vi "Restore to Defaults.vi"(6 "User interface enqueuer":refnum<class "Message Enqueuer.lvclass">, 7 "Rack Number":string, 8 "error in":errorcluster, 9 "JSON Variant Clusters":T1, 10 "JSON path cluster":T2, 11 "Part Name in":string) -> (0 "error out":errorcluster, 2 "Algo JSON variant":variant, 3 "RC JSON variant":variant)   [LabVIEW 2019, in "ZenGage v3.0 UI.lvclass"]
uses:
  ZenGage v3.0 UI.lvclass
  User Interface Messages/User Interface messages/Display Popup Msg/DisplayPopup_UI.lvclass
  Common/Controls/Pop-up Input.ctl
  <vilib>/Utility/miscctls.llb/LVPoint32TypeDef.ctl
  Type Definitions/Edit tolerance settings/Rack Selection.ctl
  <vilib>/ActorFramework/Message Enqueuer/Message Enqueuer.lvclass
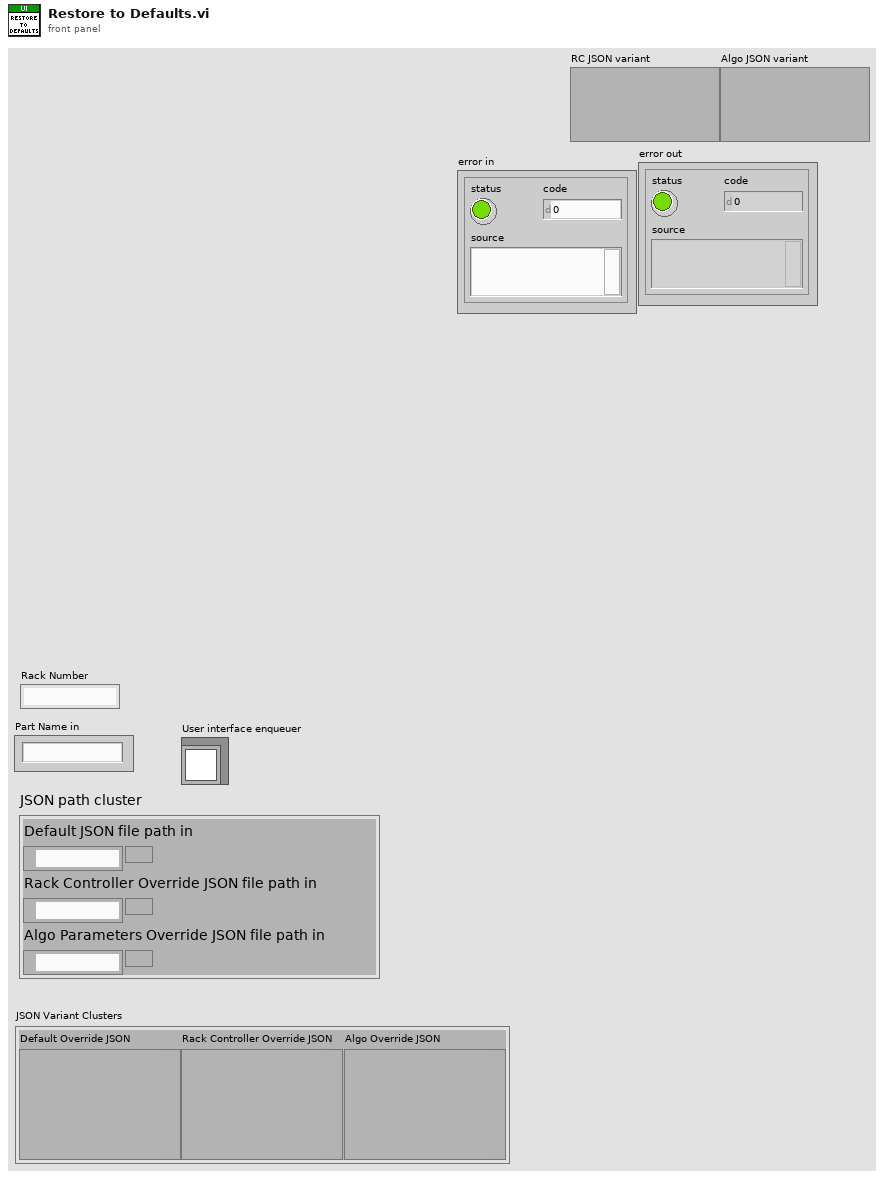
[diagram p1: front panel]
types:
  T1 = cluster{"Default Override JSON":variant, "Rack Controller Override JSON":variant, "Algo Override JSON":variant}
  T2 = cluster{"Default JSON file path in":path, "Rack Controller Override JSON file path in":path, "Algo Parameters Override JSON file path in":path}
  T3 = typedef "ZenGage v3.0 UI.lvclass/Rack Selection.ctl" = enum16{"Both Racks", "Rack 2", "Rack 1"}
  T4 = typedef "LVPoint32TypeDef.ctl" = cluster{"Horizontal":i32, "Vertical":i32}
  T5 = cluster{"Measurement Values":string[][], "Cluster of Limits":cluster{"LSL":dbl, "USL":dbl, "LCL":dbl, "UCL":dbl}, "Rack Selection":T3, "M and N Array":cluster{"M1":u64, "M2":u64, "N1":u64, "N2":u64}[], "Ticked Measurement Index":u32[], "Measurements Enabled":bool[], "Current Active Position":T4, "Current ticked measurement":dbl}
  T6 = typedef "Pop-up Input.ctl" = cluster{"Pop-up Type":enum16{"Open Logo Display", "Close Logo Display", "Open Loading Bar", "Close Loading Bar", "Open Alert Display", "Close Alert Display", "One button dialog box", "Two button dialog box", "User Authentication"}, "Title":string, "Message":string, "Button 1 Text":string, "Button 2 Text":string, "Show Close? T/F":bool, "Title Blink? T/F":bool, "Title Blink Colour":u32}
  T7 = cluster{"Measurement Values":string[][], "Enabled Disable Array":bool[]}
  T8 = cluster{"Name":string, "ImageStreams":cluster{"ThreadName":string, "RackEnable":bool, "ThreadId":dbl, "RackId":dbl, "DifferenceParameter":dbl, "SplitCameraIDs":i32[], "ImagingViews":cluster{"ViewName":string, "ViewEnable":bool, "ImageID":dbl, "CameraID":dbl, "CalibrationFilePath":string, "CalibImageFormat":string, "ReferenceCoordSystem":cluster{"Method":cluster{"Algo":string, "BaseReference":cluster{"OriginX":dbl, "OriginY":dbl, "Angle":dbl, "AxisReference":dbl}}, "ROI":cluster{"ROI":cluster{"Left":dbl, "Top":dbl, "Right":dbl, "Bottom":dbl, "Rotation":dbl}, "EdgeOptions":cluster{"EdgePolarity":dbl, "KernelSize":dbl, "Width":dbl, "MinimumEdgeStrength":dbl, "InterpolationType":dbl, "DataProcessingMethod":dbl}, "LineOptions":cluster{"NumberofLines":dbl, "Type":dbl, "MinScore":dbl, "MaxScore":dbl, "Orientation":dbl, "AngleRange":dbl, "AngleTolerance":dbl, "StepSize":dbl, "MinSNR":dbl, "MinPoints":dbl, "HoughIterations":dbl}, "Process":dbl, "StepSize":dbl, "SearchDirection":dbl, "CircleEdgeOptions":cluster{"SearchDirection":dbl, "EdgeOptions":cluster{"EdgePolarity":dbl, "KernelSize":dbl, "Width":dbl, "MinimumEdgeStrength":dbl, "InterpolationType":dbl, "DataProcessingMethod":dbl}}, "CircleFitOptions":cluster{"Process":dbl, "StepSize":dbl, "MAxPixelRadius":dbl}, "CircleSearchDirection":dbl, "CurveParameters":cluster{"ExtractionMode":dbl, "EdgeThreshold":dbl, "EdgeFilterSize":dbl, "MinLength":dbl, "RowSearchStepSize":dbl, "ColSearchStepSize":dbl, "MaxEndpointGap":dbl, "Closed":bool, "Subpixel":bool}, "MinimumMatchScore":dbl, "CircleDescriptor":cluster{"MinRadius":dbl, "MaxRadius":dbl}, "EllipseDescriptor":cluster{"MinMajorRadius":dbl, "MaxMajorRadius":dbl, "MinMinorRadius":dbl, "MaxMinorRadius":dbl}, "ParallelLines":cluster{"First":dbl, "Second":dbl, "Third":dbl}}[], "Name":string, "OverlayOptions":cluster{"OverlayEnable":bool, "OverlayText":string, "OverlayCoords":i32[], "OverlayAngle":dbl, "OverlayTextSize":dbl, "OverlayTextColor":string, "OverlayROI":bool, "OverlayRakeLine":bool, "OverlayPoints":bool}}, "CameraAngle":i32[]}[]}[], "Measurements":cluster{"RackID":dbl, "ImageID":dbl, "CameraID":dbl, "MeasurementId":dbl, "Name":string, "AlgoName":string, "Type":string, "MeasurementEnable":bool, "AlgorithmSequence":cluster{"RefernceEdge":cluster{"Enable":bool, "Method":string, "RefROI":cluster{"Left":dbl, "Top":dbl, "Right":dbl, "Bottom":dbl, "Rotation":dbl}, "EdgeOptions":cluster{"EdgePoarity":dbl, "KernelSize":dbl, "Width":dbl, "MinimumEdgeStrength":dbl, "InterpolationType":dbl, "DataProcessingMethod":dbl}, "LineOptions":cluster{"NumberofLines":dbl, "Type":dbl, "MinScore":dbl, "MaxScore":dbl, "Orientation":dbl, "AngleRange":dbl, "AngleTolerance":dbl, "StepSize":dbl, "MinSNR":dbl, "MinPoints":dbl, "HoughIterations":dbl}, "SearchDirection":dbl}, "Measurement":cluster{"ROI1":cluster{"Enable":bool, "ROI":cluster{"Left":dbl, "Top":dbl, "Right":dbl, "Bottom":dbl, "Rotation":dbl}, "EdgeOptions":cluster{"EdgePoarity":dbl, "KernelSize":dbl, "Width":dbl, "MinimumEdgeStrength":dbl, "InterpolationType":dbl, "DataProcessingMethod":dbl}, "LineOptions":cluster{"NumberofLines":dbl, "Type":dbl, "MinScore":dbl, "MaxScore":dbl, "Orientation":dbl, "AngleRange":dbl, "AngleTolerance":dbl, "StepSize":dbl, "MinSNR":dbl, "MinPoints":dbl, "HoughIterations":dbl}, "Process":dbl, "StepSize":dbl, "SearchDirection":dbl, "CircleEdgeOptions":cluster{"SearchDirection":dbl, "EdgeOptions":cluster{"EdgePoarity":dbl, "KernelSize":dbl, "Width":dbl, "MinimumEdgeStrength":dbl, "InterpolationType":dbl, "DataProcessingMethod":dbl}}, "CircleFitOptions":cluster{"Process":dbl, "StepSize":dbl, "MAxPixelRadius":dbl}, "CircleSearchDirection":dbl, "CurveParameters":cluster{"ExtractionMode":dbl, "EdgeThreshold":dbl, "EdgeFilterSize":dbl, "MinLength":dbl, "RowSearchStepSize":dbl, "ColSearchStepSize":dbl, "MaxEndpointGap":dbl, "Closed":bool, "Subpixel":bool}, "MinimumMatchScore":dbl, "CircleDescriptor":cluster{"MinRadius":dbl, "MaxRadius":dbl}, "EllipseDescriptor":cluster{"MinMajorRadius":dbl, "MaxMajorRadius":dbl, "MinMinorRadius":dbl, "MaxMinorRadius":dbl}}, "ROI2":cluster{"Enable":bool, "ROI":cluster{"Left":dbl, "Top":dbl, "Right":dbl, "Bottom":dbl, "Rotation":dbl}, "EdgeOptions":cluster{"EdgePoarity":dbl, "KernelSize":dbl, "Width":dbl, "MinimumEdgeStrength":dbl, "InterpolationType":dbl, "DataProcessingMethod":dbl}, "LineOptions":cluster{"NumberofLines":dbl, "Type":dbl, "MinScore":dbl, "MaxScore":dbl, "Orientation":dbl, "AngleRange":dbl, "AngleTolerance":dbl, "StepSize":dbl, "MinSNR":dbl, "MinPoints":dbl, "HoughIterations":dbl}, "Process":dbl, "StepSize":dbl, "SearchDirection":dbl, "CircleEdgeOptions":cluster{"SearchDirection":dbl, "EdgeOptions":cluster{"EdgePoarity":dbl, "KernelSize":dbl, "Width":dbl, "MinimumEdgeStrength":dbl, "InterpolationType":dbl, "DataProcessingMethod":dbl}}, "CircleFitOptions":cluster{"Process":dbl, "StepSize":dbl, "MAxPixelRadius":dbl}, "CircleSearchDirection":dbl, "CurveParameters":cluster{"ExtractionMode":dbl, "EdgeThreshold":dbl, "EdgeFilterSize":dbl, "MinLength":dbl, "RowSearchStepSize":dbl, "ColSearchStepSize":dbl, "MaxEndpointGap":dbl, "Closed":bool, "Subpixel":bool}, "MinimumMatchScore":dbl, "CircleDescriptor":cluster{"MinRadius":dbl, "MaxRadius":dbl}, "EllipseDescriptor":cluster{"MinMajorRadius":dbl, "MaxMajorRadius":dbl, "MinMinorRadius":dbl, "MaxMinorRadius":dbl}}}}, "MathExpression":cluster{"Algorithm":string, "MathExpression":string, "ResultVariable":string}, "MathCorrectionParameters":cluster{"Radius":dbl, "CurlGap":dbl, "Thickness":dbl, "MeasurementIndices":i32[], "MathAlgoName":string, "MathAlgoFormula":string, "CorrectionForAngle":i32[], "NumericAray":i32[], "StringArray":string[]}, "ResultVariableCluster":cluster{"RVName":string, "RVSequence":string, "RVIndex":dbl, "RVID":dbl, "RVValue":dbl}, "CalibrationCoefficients":cluster{"A1":dbl, "A2":dbl, "A3":dbl}, "UserCalibCoefficients":cluster{"UserCorrectionLinearityCoeff":dbl, "UserCorrectionBiasCoeff":dbl}, "SpecValues":cluster{"LCL":dbl, "UCL":dbl, "LSL":dbl, "USL":dbl, "NominalValue":dbl}, "OverlayOptions":cluster{"OverlayEnable":bool, "OverlayText":string, "OverlayCoords":i32[], "OverlayAngle":dbl, "OverlayTextSize":dbl, "OverlayTextColor":string, "OverlayROI":bool, "OverlayRakeLine":bool, "OverlayPoints":bool}, "DatalogEnable":bool, "DisplayIcon":string}[]}
  T9 = cluster{"RackID":dbl, "ImageID":dbl, "CameraID":dbl, "MeasurementId":dbl, "Name":string, "AlgoName":string, "Type":string, "MeasurementEnable":bool, "AlgorithmSequence":cluster{"RefernceEdge":cluster{"Enable":bool, "Method":string, "RefROI":cluster{"Left":dbl, "Top":dbl, "Right":dbl, "Bottom":dbl, "Rotation":dbl}, "EdgeOptions":cluster{"EdgePoarity":dbl, "KernelSize":dbl, "Width":dbl, "MinimumEdgeStrength":dbl, "InterpolationType":dbl, "DataProcessingMethod":dbl}, "LineOptions":cluster{"NumberofLines":dbl, "Type":dbl, "MinScore":dbl, "MaxScore":dbl, "Orientation":dbl, "AngleRange":dbl, "AngleTolerance":dbl, "StepSize":dbl, "MinSNR":dbl, "MinPoints":dbl, "HoughIterations":dbl}, "SearchDirection":dbl}, "Measurement":cluster{"ROI1":cluster{"Enable":bool, "ROI":cluster{"Left":dbl, "Top":dbl, "Right":dbl, "Bottom":dbl, "Rotation":dbl}, "EdgeOptions":cluster{"EdgePoarity":dbl, "KernelSize":dbl, "Width":dbl, "MinimumEdgeStrength":dbl, "InterpolationType":dbl, "DataProcessingMethod":dbl}, "LineOptions":cluster{"NumberofLines":dbl, "Type":dbl, "MinScore":dbl, "MaxScore":dbl, "Orientation":dbl, "AngleRange":dbl, "AngleTolerance":dbl, "StepSize":dbl, "MinSNR":dbl, "MinPoints":dbl, "HoughIterations":dbl}, "Process":dbl, "StepSize":dbl, "SearchDirection":dbl, "CircleEdgeOptions":cluster{"SearchDirection":dbl, "EdgeOptions":cluster{"EdgePoarity":dbl, "KernelSize":dbl, "Width":dbl, "MinimumEdgeStrength":dbl, "InterpolationType":dbl, "DataProcessingMethod":dbl}}, "CircleFitOptions":cluster{"Process":dbl, "StepSize":dbl, "MAxPixelRadius":dbl}, "CircleSearchDirection":dbl, "CurveParameters":cluster{"ExtractionMode":dbl, "EdgeThreshold":dbl, "EdgeFilterSize":dbl, "MinLength":dbl, "RowSearchStepSize":dbl, "ColSearchStepSize":dbl, "MaxEndpointGap":dbl, "Closed":bool, "Subpixel":bool}, "MinimumMatchScore":dbl, "CircleDescriptor":cluster{"MinRadius":dbl, "MaxRadius":dbl}, "EllipseDescriptor":cluster{"MinMajorRadius":dbl, "MaxMajorRadius":dbl, "MinMinorRadius":dbl, "MaxMinorRadius":dbl}}, "ROI2":cluster{"Enable":bool, "ROI":cluster{"Left":dbl, "Top":dbl, "Right":dbl, "Bottom":dbl, "Rotation":dbl}, "EdgeOptions":cluster{"EdgePoarity":dbl, "KernelSize":dbl, "Width":dbl, "MinimumEdgeStrength":dbl, "InterpolationType":dbl, "DataProcessingMethod":dbl}, "LineOptions":cluster{"NumberofLines":dbl, "Type":dbl, "MinScore":dbl, "MaxScore":dbl, "Orientation":dbl, "AngleRange":dbl, "AngleTolerance":dbl, "StepSize":dbl, "MinSNR":dbl, "MinPoints":dbl, "HoughIterations":dbl}, "Process":dbl, "StepSize":dbl, "SearchDirection":dbl, "CircleEdgeOptions":cluster{"SearchDirection":dbl, "EdgeOptions":cluster{"EdgePoarity":dbl, "KernelSize":dbl, "Width":dbl, "MinimumEdgeStrength":dbl, "InterpolationType":dbl, "DataProcessingMethod":dbl}}, "CircleFitOptions":cluster{"Process":dbl, "StepSize":dbl, "MAxPixelRadius":dbl}, "CircleSearchDirection":dbl, "CurveParameters":cluster{"ExtractionMode":dbl, "EdgeThreshold":dbl, "EdgeFilterSize":dbl, "MinLength":dbl, "RowSearchStepSize":dbl, "ColSearchStepSize":dbl, "MaxEndpointGap":dbl, "Closed":bool, "Subpixel":bool}, "MinimumMatchScore":dbl, "CircleDescriptor":cluster{"MinRadius":dbl, "MaxRadius":dbl}, "EllipseDescriptor":cluster{"MinMajorRadius":dbl, "MaxMajorRadius":dbl, "MinMinorRadius":dbl, "MaxMinorRadius":dbl}}}}, "MathExpression":cluster{"Algorithm":string, "MathExpression":string, "ResultVariable":string}, "MathCorrectionParameters":cluster{"Radius":dbl, "CurlGap":dbl, "Thickness":dbl, "MeasurementIndices":i32[], "MathAlgoName":string, "MathAlgoFormula":string, "CorrectionForAngle":i32[], "NumericAray":i32[], "StringArray":string[]}, "ResultVariableCluster":cluster{"RVName":string, "RVSequence":string, "RVIndex":dbl, "RVID":dbl, "RVValue":dbl}, "CalibrationCoefficients":cluster{"A1":dbl, "A2":dbl, "A3":dbl}, "UserCalibCoefficients":cluster{"UserCorrectionLinearityCoeff":dbl, "UserCorrectionBiasCoeff":dbl}, "SpecValues":cluster{"LCL":dbl, "UCL":dbl, "LSL":dbl, "USL":dbl, "NominalValue":dbl}, "OverlayOptions":cluster{"OverlayEnable":bool, "OverlayText":string, "OverlayCoords":i32[], "OverlayAngle":dbl, "OverlayTextSize":dbl, "OverlayTextColor":string, "OverlayROI":bool, "OverlayRakeLine":bool, "OverlayPoints":bool}, "DatalogEnable":bool, "DisplayIcon":string}[]
  T10 = typedef "ZenGage v3.0 UI.lvclass/Edit Tolerance Input.ctl" = cluster{"Measurement Values":string[][], "Cluster of Limits":cluster{"LSL":dbl, "USL":dbl, "LCL":dbl, "UCL":dbl}, "Rack Selection":T3, "M and N Array":cluster{"M1":u64, "M2":u64, "N1":u64, "N2":u64}[], "Ticked Measurement Index":u32[], "Measurements Enabled":bool[], "Current Active Position":T4, "Current ticked measurement":dbl}
  T11 = cluster{"M1":u64, "M2":u64, "N1":u64, "N2":u64}[]
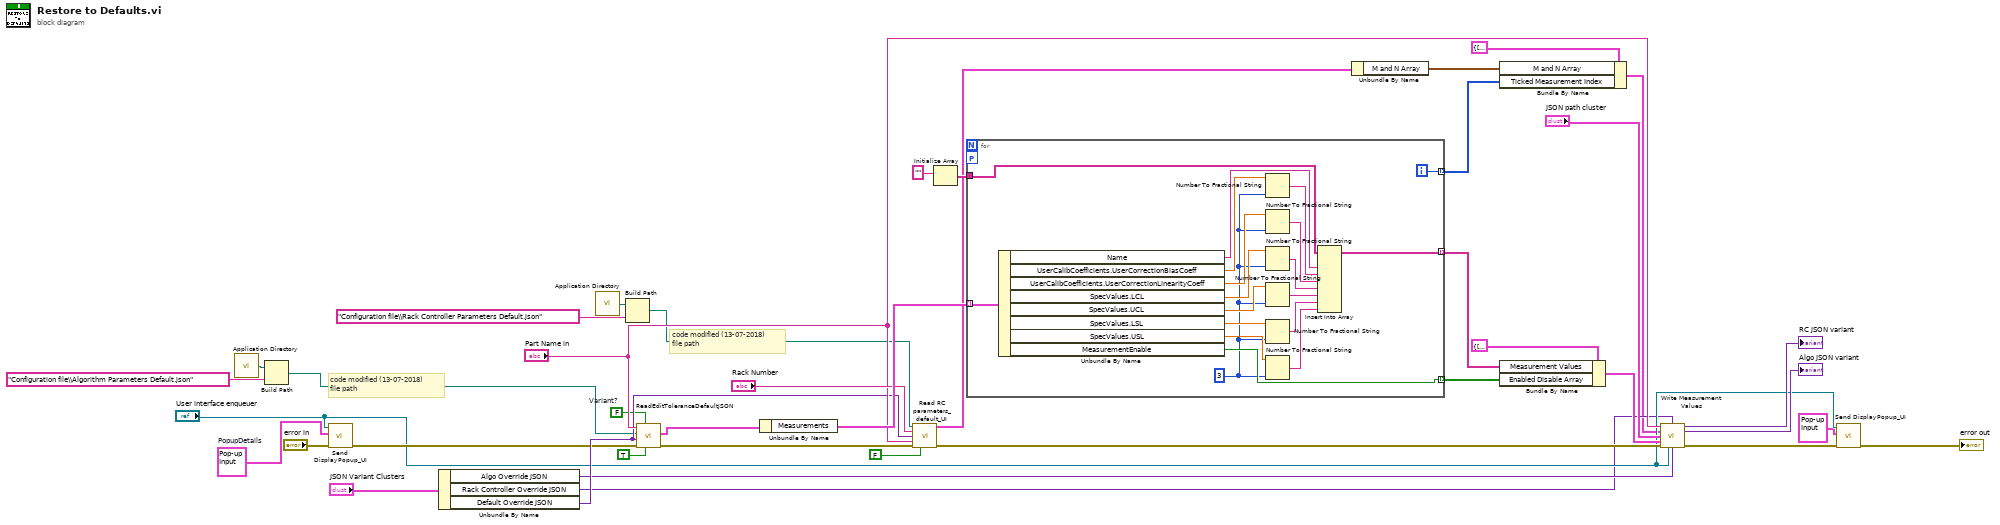
[diagram p0: block diagram]
diagram:
  w10 = T6 {"Pop-up Type"=enum."Open Loading Bar", "Title"="", "Message"="Reading default parameters...", "Button 1 Text"="", "Button 2 Text"="", "Show Close? T/F"=FALSE, "Title Blink? T/F"=FALSE, "Title Blink Colour"=0}  # PopupDetails
  w27 = FALSE  # Variant?
  # "code modified (13-07-2018)\nfile path"
  # "code modified (13-07-2018)\nfile path"
  n1 = call <vilib>:"Application Directory.vi"() -> ("Application Directory"=w23:path)
  n2 = Build Path(base path=w23, name or relative path="Configuration file\\Algorithm Parameters Default.json") -> (appended path=w21:path)
  n3 = call "Send DisplayPopup_UI.vi"("error in (no error)"="error in", "PopupDetails"=w10, "Message Enqueuer"="User interface enqueuer") -> ("error out"=w16:errorcluster)  [unwired: 7 in, 1 out]
  n4 = Unbundle By Name("JSON Variant Clusters") -> ("Algo Override JSON"=w8:variant, "Rack Controller Override JSON"=w7:variant, "Default Override JSON"=w30:variant)
  n5 = call <vilib>:"Application Directory.vi"() -> ("Application Directory"=w20:path)
  n6 = Build Path(base path=w20, name or relative path="Configuration file\\Rack Controller Parameters Default.json") -> (appended path=w19:path)
  n7 = call "ReadEditToleranceDefaultJSON.vi"("Default?"=TRUE, "Variant?"=w27, "error in"=w16, "Default JSON Variant in"=w30, "Read Edit Tolerance \nOverride JSON"=w21, "Part Name"="Part Name in") -> ("error out"=w15:errorcluster, "Algo parameters"=w1:T8)  [unwired: 3 in, 1 out]
  n8 = Unbundle By Name(w1) -> ("Measurements"=w40:T9)
  n9 = call "Read RC parameters_default_UI.vi"("JSON FilePath"=w19, "Rack Id"="Rack Number", "Variant"=w30, "Part Name"="Part Name in", "error in (no error)"=w15, "Variant?"=FALSE) -> ("Output Edit Tolerance cluster"=w28:T10, "error out"=w14:errorcluster)  [unwired: 7 in, 1 out]
  n10 = Initialize Array("") -> (w38:string[])  [unwired: 1 in]
  n11 = for {
    tunnel: w40 -> [w59] mode=indexing
    tunnel: w38 -> [w55]
    tunnel: [w56] -> w35 mode=indexing
    tunnel: [w54] -> w4 mode=indexing
    tunnel: [w53] -> w32 mode=indexing
    workers-P: _ -> [_]
    i -> [w54]
    w47 = i16 3 ("width (-)")
    n12 = Unbundle By Name(w59) -> ("Name"=w57:string, "UserCalibCoefficients.UserCorrectionBiasCoeff"=w58:dbl, "UserCalibCoefficients.UserCorrectionLinearityCoeff"=w52:dbl, "SpecValues.LCL"=w51:dbl, "SpecValues.UCL"=w50:dbl, "SpecValues.LSL"=w49:dbl, "SpecValues.USL"=w48:dbl, "MeasurementEnable"=w53:bool)
    n13 = Number To Fractional String(number=w58, precision (6)=w47) -> (F-format string=w46:string)  [unwired: 2 in]
    n14 = Number To Fractional String(number=w52, precision (6)=w47) -> (F-format string=w45:string)  [unwired: 2 in]
    n15 = Number To Fractional String(number=w51, precision (6)=w47) -> (F-format string=w44:string)  [unwired: 2 in]
    n16 = Number To Fractional String(number=w50, precision (6)=w47) -> (F-format string=w43:string)  [unwired: 2 in]
    n17 = Number To Fractional String(number=w49, precision (6)=w47) -> (F-format string=w42:string)  [unwired: 2 in]
    n18 = Number To Fractional String(number=w48, precision (6)=w47) -> (F-format string=w41:string)  [unwired: 2 in]
    n19 = Insert Into Array(array=w55, new element #1=w57, new element #2=w46, new element #3=w45, new element #4=w44, new element #5=w43, new element #6=w42, new element #7=w41) -> (w56:string[])  [unwired: 1 in]
  }
  n20 = Unbundle By Name(w28) -> ("M and N Array"=w5:T11)
  n21 = Bundle By Name(cluster=T5 {"Measurement Values"=[], "Cluster of Limits"={"LSL"=0.0, "USL"=0.0, "LCL"=0.0, "UCL"=0.0}, "Rack Selection"=enum."Both Racks", "M and N Array"=[], "Ticked Measurement Index"=[], "Measurements Enabled"=[], "Current Active Position"={"Horizontal"=0, "Vertical"=0}, "Current ticked measurement"=0.0} ("Input Data Cluster"), "M and N Array"=w5, "Ticked Measurement Index"=w4) -> (w3:T5)
  n22 = Bundle By Name(cluster=T7 {"Measurement Values"=[["W", "AET", "2.5", "-10", "100", "-10", "100", "1", "0"], ["H", "TT Width", "3.225", "2", "20", "-10", "100", "1", "0"]], "Enabled Disable Array"=[TRUE, FALSE]} ("Measurements Cluster"), "Measurement Values"=w35, "Enabled Disable Array"=w32) -> (w34:T7)
  n23 = call "Write Measurement Values.vi"("Selected Part Name"="Part Name in", "RC JSON variant in"=w7, "Input Data Cluster"=w3, "Input File Paths Cluster"="JSON path cluster", "Measurements Cluster"=w34, "error in"=w14, "User interface enqueuer"="User interface enqueuer", "Algo JSON variant in"=w8) -> ("RC JSON variant out"=→"RC JSON variant":variant, "Algo JSON variant out"=→"Algo JSON variant":variant, "error out"=w13:errorcluster)  [unwired: 5 in]
  n24 = call "Send DisplayPopup_UI.vi"("error in (no error)"=w13, "PopupDetails"=T6 {"Pop-up Type"=enum."Close Loading Bar", "Title"="", "Message"="", "Button 1 Text"="", "Button 2 Text"="", "Show Close? T/F"=FALSE, "Title Blink? T/F"=FALSE, "Title Blink Colour"=0}, "Message Enqueuer"="User interface enqueuer") -> ("error out"=→"error out":errorcluster)  [unwired: 7 in, 1 out]
